vi "Adresse Alarme.vi"(8 "error in (no error)":errorcluster caption="Fehler (Eingang, kein Fehler)", 11 "mini8 Steuerung PNS Eingang":refnum<class "mini8 Steuerung PNS.lvclass">) -> (0 "error out":errorcluster caption="Fehler (Ausgang)", 2 "Adressen":T1, 3 "mini8 Steuerung PNS Ausgang":refnum<class "mini8 Steuerung PNS.lvclass">)   [LabVIEW 2020, in "mini8 Steuerung PNS.lvclass"]
uses:
  mini8 Steuerung PNS.lvclass
  D:/LabView_2020/LP und Compact Standardprogramm_20-10-14/ObjektKlassen/Steuerung PNS/Steuerung PNS.lvclass
  Adresse.ctl
  AdressIndex.ctl
  Steuerung PNS.lvclass
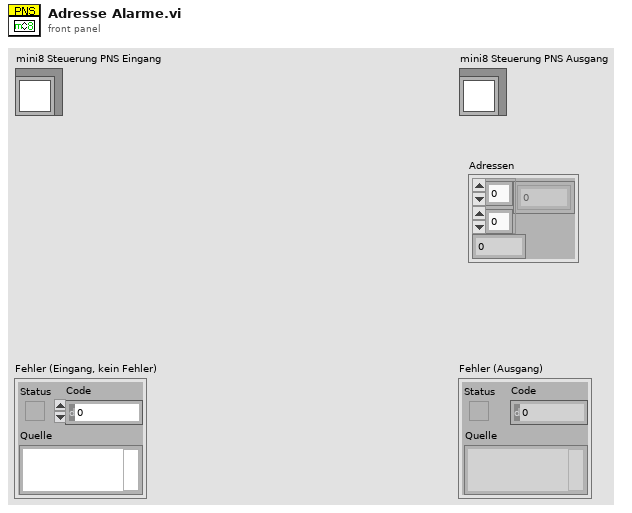
[diagram p1: front panel]
types:
  T1 = typedef "Steuerung PNS.lvclass/Adresse.ctl" = cluster{i32[][], i32}
  T2 = typedef "Steuerung PNS.lvclass/AdressIndex.ctl" = cluster{"Index":i32, "Index 2":i32, "Länge2":i32, "\nAnzahl":i32}
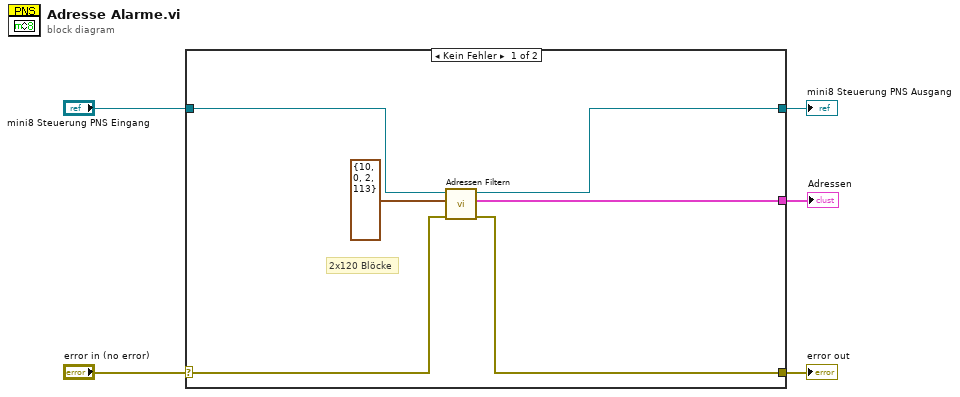
[diagram p0: block diagram]
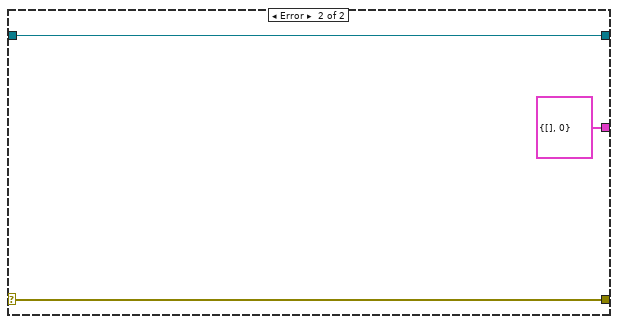
[diagram p2: hidden frame]
diagram:
  n1 = case shown="Kein Fehler" "error in (no error)" {
    selector: "error in (no error)" -> [w7 w14]
    tunnel: [w6 w14] -> w4
    tunnel: [w8 w13] -> w2
    tunnel: "mini8 Steuerung PNS Eingang" -> [w9 w13]
    tunnel: [w10 cluster{i32[][], i32} {[], 0} ("Adressen")] -> w1
    frame No Error {
      # "2x120 Blöcke"
      n2 = call "Adressen Filtern.vi"("error in (no error)"=w7, "AdressIndex"=T2 {"Index"=10, "Index 2"=0, "Länge2"=2, "\nAnzahl"=113}, "Steuerung PNS Eingang"=w9) -> ("error out"=w6:errorcluster, "Adressen"=w10:cluster{i32[][], i32}, "Steuerung PNS Ausgang"=w8:refnum<class "mini8 Steuerung PNS.lvclass">)  [unwired: 6 in]
    }
    frame Error {
    }
  }
  "error out" <- w4
  "mini8 Steuerung PNS Ausgang" <- w2
  "Adressen" <- w1
